vi "gas monitor.vi"() -> ()   [LabVIEW 2021]
uses:
  <vilib>/MakerHub/LINX/Public/Peripherals/Analog/Analog Read 1 Chan.vi
  <vilib>/MakerHub/LINX/Public/Peripherals/Digital/Digital Write 1 Chan.vi
  <vilib>/MakerHub/LINX/Public/Peripherals/Analog/Analog Read N Chans.vi
  <vilib>/MakerHub/LINX/Public/Peripherals/Digital/Digital Write N Chans.vi
  <vilib>/MakerHub/LINX/Private/Local IO/LinxAnalogRead.vi
  <vilib>/MakerHub/LINX/Public/Utilities/Check Channel.vi
  <vilib>/MakerHub/LINX/Private/Local IO/LinxDigitalWrite.vi
  <vilib>/MakerHub/LINX/Public/Utilities/Open Serial.vi
  <vilib>/MakerHub/LINX/Public/Sensors/Motion/Servo/Servo Open One Channel.vi
  <vilib>/MakerHub/LINX/Private/Utilties/Generate Error.vi
  <vilib>/MakerHub/LINX/Public/Sensors/Motion/Servo/Servo Set Pulse Width One Channel.vi
  <vilib>/MakerHub/LINX/Public/Sensors/Motion/Servo/Servo Close One Channel.vi
  <vilib>/MakerHub/LINX/LMH-LINX.lvlib
  <vilib>/MakerHub/LINX/Public/Sensors/Motion/Servo/Servo.lvlib
  <vilib>/Analysis/NI_AALPro.lvlib
panel:
  in  "Serial Port":refnum<visa-resource-name>="N/A"
  in  "Gas Value":dbl
  out "Gas Output":dbl
  in  "stop":bool
  # "Gas Concentration Regulator"
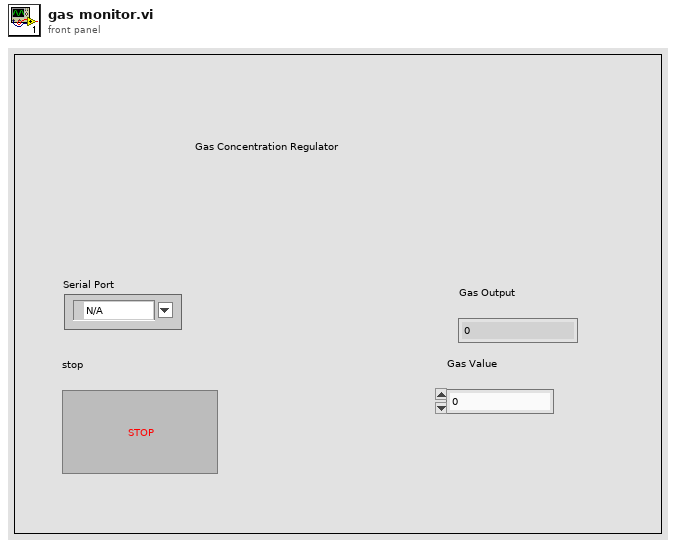
[diagram p1: front panel]
types:
  T1 = typedef "LMH-LINX.lvlib/LINX Ref.ctl" = cluster{"IO":T2, "Interface":T3, "LINX Device Config":T4}
  T2 = typedef "LMH-LINX.lvlib/Platform.ctl" = enum16{"Remote", "Local"}
  T3 = typedef "LMH-LINX.lvlib/Interface.ctl" = enum16{"Serial", "TCP"}
  T4 = typedef "LMH-LINX.lvlib/Device.lvlib/LINX Device Config.ctl" = cluster{"Interface":T3, "COM Port":refnum<visa-resource-name>, "TCP Configuration":T5, "Device Family":u8, "Device ID":u8, "Device Name":string, "TCP Ref":refnum<k5>, "Channels":T6}
  T5 = typedef "LMH-LINX.lvlib/Device.lvlib/TCP Config.ctl" = cluster{"IP Address":string, "Port":u16}
  T6 = typedef "LMH-LINX.lvlib/Channels.ctl" = cluster{"DI":u8[], "DO":u8[], "AI":u8[], "AO":u8[], "PWM":u8[], "QE":u8[], "UART":u8[], "I2C 2":u8[], "SPI":u8[], "CAN":u8[], "Servo":u8[], "AI Ref (V)":dbl, "AI Resolution (Bits)":u8, "AO Ref (V)":dbl, "AO Resolution (Bits)":u8}
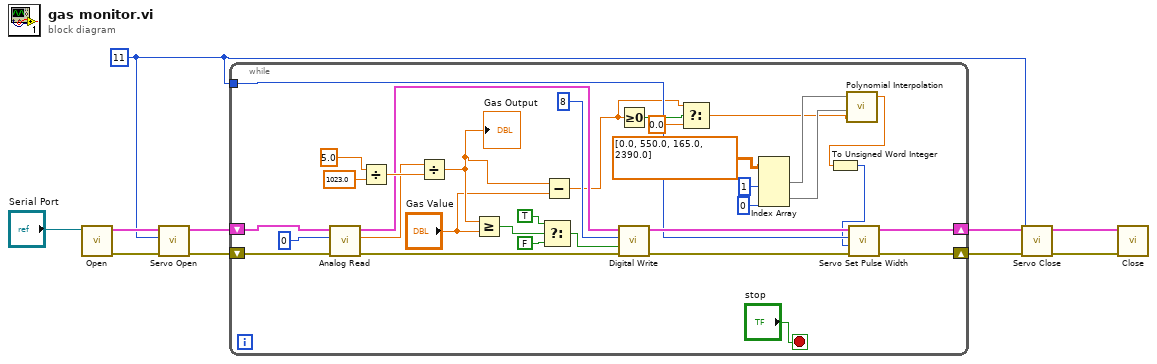
[diagram p0: block diagram]
diagram:
  w1 = u8 11 ("Servo Channel")
  n1 = call-poly <vilib>:"Open.vi"("Serial Port"="Serial Port") -> ("Error Out"=w2:errorcluster, "LINX Resource"=w3:T1)  [unwired: 8 in, 1 out]
  n2 = call-poly <vilib>:"Servo Open.vi"("Error In"=w2, "Servo Channel"=w1, "LINX Resource"=w3) -> ("Error Out"=w4:errorcluster, "LINX Resource"=w5:T1)  [unwired: 7 in]
  n3 = while {
    shift-right: [w28] -> w9
    shift-left: w5 -> [w35]
    shift-right: [w27] -> w7
    shift-left: w4 -> [w34]
    tunnel: w1 -> [w24]
    stop <- "stop" stop-if-true
    n4 = call-poly <vilib>:"Analog Read.vi"("Error In"=w34, "Analog Channel"=u8 0, "LINX Resource"=w35) -> ("Error Out"=w31:errorcluster, "Voltage"=w30:dbl, "LINX Resource"=w32:T1)  [unwired: 5 in, 1 out]
    n5 = Divide(x=5.0, y=1023.0) -> (x/y=w42:dbl)
    n6 = Divide(x=w30, y=w42) -> (x/y=w18:dbl)
    "Gas Output" <- w18
    n7 = Greater Or Equal?(x=w18, y="Gas Value") -> (x >= y?=w39:bool)
    n8 = Select(t=TRUE, s=w39, f=FALSE) -> (s? t:f=w29:bool)
    n9 = Subtract(x=w18, y="Gas Value") -> (x-y=w14:dbl)
    n10 = Greater Or Equal To 0?(x=w14) -> (x >= 0?=w13:bool)
    n11 = call-poly <vilib>:"Digital Write.vi"("Error In"=w31, "Output Value"=w29, "DO Channel"=u8 8, "LINX Resource"=w32) -> ("Error Out"=w25:errorcluster, "LINX Resource"=w26:T1)  [unwired: 6 in]
    n12 = Select(t=w14, s=w13, f=0.0) -> (s? t:f=w11:dbl)
    n13 = Index Array(array=dbl[][] [[0.0, 550.0], [165.0, 2390.0]], index (col) #1=1 ("disabled index (col)"), index (col) #2=0 ("index (col)")) -> (element #1=w20:dbl[], element #2=w19:dbl[])  [unwired: 2 in]
    n14 = call <vilib>:"Polynomial Interpolation.vi"("x value"=w11, "X"=w19, "Y"=w20) -> ("interpolation value"=w22:dbl)  [unwired: 2 out]
    n15 = To Unsigned Word Integer(number=w22) -> (unsigned 16bit integer=w23:u16)
    n16 = call-poly <vilib>:"Servo Set Pulse Width.vi"("Error In"=w25, "Pulse Width (uS)"=w23, "Servo Channel"=w24, "LINX Resource"=w26) -> ("Error Out"=w27:errorcluster, "LINX Resource"=w28:T1)  [unwired: 6 in]
  }
  n17 = call-poly <vilib>:"Servo Close.vi"("Error In"=w7, "Servo Channel"=w1, "LINX Resource"=w9) -> ("Error Out"=w6:errorcluster, "LINX Resource"=w8:T1)  [unwired: 7 in]
  n18 = call <vilib>:"Close.vi"("Error In"=w6, "LINX Resource"=w8) -> ()  [unwired: 9 in, 1 out]
